vi "insertBuffer.vi"(1 "data":string, 2 "array":string[](array[string])) -> (0 "output array":string[](array[string]))   [LabVIEW 2019]
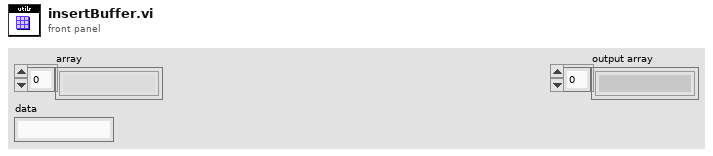
[diagram p1: front panel]
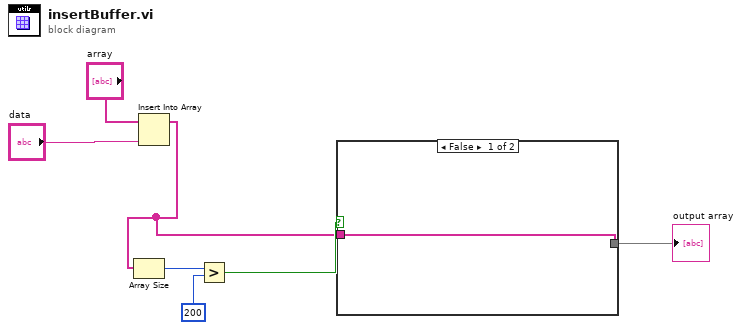
[diagram p0: block diagram]
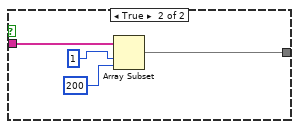
[diagram p2: hidden frame]
diagram:
  n1 = Insert Into Array(array="array", new element="data") -> (w2:string[])  [unwired: 1 in]
  n2 = Array Size(array=w2) -> (size(s)=w6:i32)
  n3 = Greater?(x=w6, y=200) -> (0:w3:bool)
  n4 = case shown="False" w3 {
    tunnel: w2 -> [w8 w12]
    tunnel: [w8 w9] -> w1
    frame False {
    }
    frame True {
      n5 = Array Subset(array=w12, index=1, length=200) -> (w9:string[])
    }
  }
  "output array" <- w1
